vi "CSM Invalid Name Error.vi"(8 "error in (no error)":errorcluster, 10 "Occured":bool=TRUE, 11 "Name (\"\" to Use UUID)":string) -> (0 "error out":errorcluster)   [LabVIEW 2017, in "Communicable State Machine.lvlib"]
uses:
  Communicable State Machine.lvlib
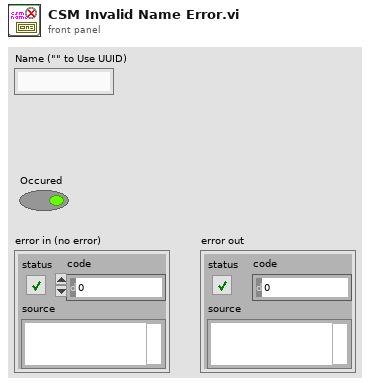
[diagram p1: front panel]
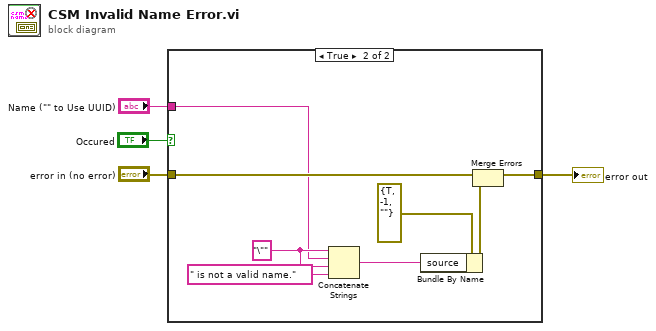
[diagram p0: block diagram]
diagram:
  n1 = case shown="True" "Occured" {
    tunnel: "error in (no error)" -> [w5 w13]
    tunnel: [w5 w12] -> w2
    tunnel: "Name (\"\" to Use UUID)" -> [_ w9]
    frame False {
    }
    frame True {
      w10 = "\"" ("string")
      n2 = Concatenate Strings(w10, w9, w10, " is not a valid name." ("string")) -> (w6:string)
      n3 = Bundle By Name(cluster=errorcluster {"status"=TRUE, "code"=-1, "source"=""} ("error in"), "source"=w6) -> (w7:errorcluster)
      n4 = Merge Errors(w13, w7) -> (w12:errorcluster)
    }
  }
  "error out" <- w2
